vi "Write OffsetDef.lvclass.vi"(8 "error in (no error)":errorcluster, 10 "OffsetDef.lvclass":refnum<class "OffsetDef.lvclass">, 11 "Offset.lvclass in":refnum<class "Offset.lvclass">) -> (0 "error out":errorcluster, 3 "Offset.lvclass out":refnum<class "Offset.lvclass">)   [LabVIEW 2014, in "TCSDataDefinitions.lvlib" / "TCSCommand.lvlib" / "OffsetCommands.lvlib" / "Offset.lvclass"]
uses:
  Offset.lvclass
  OffsetDef/OffsetDef/OffsetDef.lvclass
  Offset.lvclass/Offset.ctl
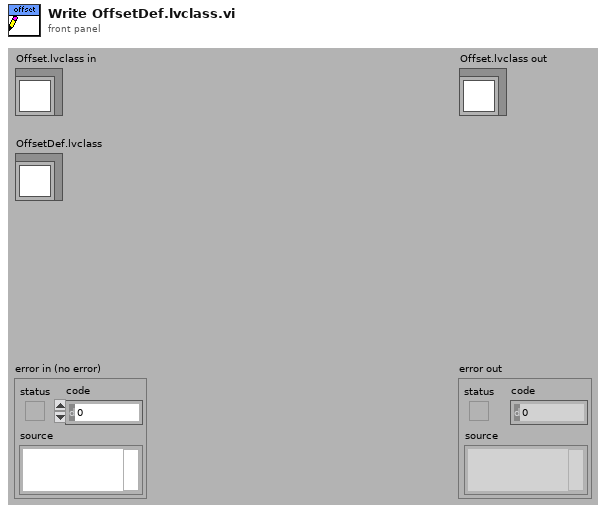
[diagram p1: front panel]
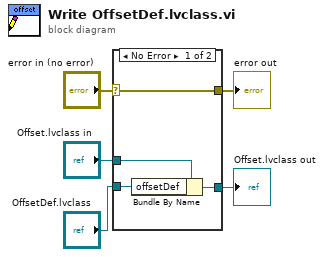
[diagram p0: block diagram]
diagram:
  n1 = case shown="No Error" "error in (no error)" {
    selector: "error in (no error)" -> [w9 w10]
    tunnel: [w9 w10] -> w4
    tunnel: [w7 w11] -> w2
    tunnel: "Offset.lvclass in" -> [w8 w11]
    tunnel: "OffsetDef.lvclass" -> [w6 _]
    frame No Error {
      n2 = Bundle By Name(cluster=w8, "offsetDef"=w6) -> (w7:refnum<class "Offset.lvclass">)
    }
    frame Error {
    }
  }
  "error out" <- w4
  "Offset.lvclass out" <- w2
